vi "Calculate Galvo Control Voltage to Image Size and Max FOV.vi"(8 "Error In":errorcluster, 11 "System Parameters [In]":T1={"Optical /HW Parameters"={"Focal Length [mm]"=0.0, "Scan Lens EFL[mm]"=0.0, "Tube Lens EFL[mm]"=0.0, "Galvo V Range (+/-)"=0.0, "Galvo Max Half Angle [Deg]"=0.0, "Max Galvo Range[%]"=0.0}, "Vibratome"={"Z Bottom [mm]"=0.0, "Pre Cut Dwell [s]"=0.0, "Blade Frequency [RPM]"=0, "Slice Speed [mm/s]"=0.0, "Post Cut Dwell [s]"=0.0, "Ramp Time [s]"=0.0, "Start X [mm]"=0.0, "Start Y [mm]"=0.0, "Slice Length [mm]"=0.0, "Slice Axis"=enum."Y Axis", "Controller VISA Ref"="COM4"}, "Table Stages"={"X Stage"={"Position"=0.0, "Is.Enabled?"=FALSE, "Is.Connected?"=FALSE, "Device SN"="45876539", "AccelerationMaximum"=0.0, "VelocityMaximum"=0.0, "Acceleration"=0.0, "Velocity"=0.0, "waitTimeout (ms)"=0, "Model"=enum."None", "Is.Homed?"=FALSE}, "Y Stage"={"Position"=0.0, "Is.Enabled?"=FALSE, "Is.Connected?"=FALSE, "Device SN"="45876539", "AccelerationMaximum"=0.0, "VelocityMaximum"=0.0, "Acceleration"=0.0, "Velocity"=0.0, "waitTimeout (ms)"=0, "Model"=enum."None", "Is.Homed?"=FALSE}, "Z Stage"={"Position"=0.0, "Is.Enabled?"=FALSE, "Is.Connected?"=FALSE, "Device SN"="45876539", "AccelerationMaximum"=0.0, "VelocityMaximum"=0.0, "Acceleration"=0.0, "Velocity"=0.0, "waitTimeout (ms)"=0, "Model"=enum."None", "Is.Homed?"=FALSE}}, "Imaging Parameter"={"Raster Scan Direction"=enum."Uni Directional", "Pixel Dwell Time [Clock Cycles]"=0, "Flyback Time [Clock Cycles]"=0, "XY Center [um]"={"X"=1.0, "Y"=1.0}, "Pixel Step Size [um]"=1.0, "XY Image Resolution"=enum."256 x 256", "Custom"=FALSE, "Custom Size"={"X"=1, "Y"=1}, "Line Averages"=1}} {"Imaging Parameter"."Line Averages" min=1 max=30 step=1; "Imaging Parameter"."Flyback Time [Clock Cycles]" max=10 step=1; "Imaging Parameter"."Pixel Step Size [um]" min=0.0 max=10.0 step=0.01; "Imaging Parameter"."Custom Size"."Y" min=1 max=30 step=1; "Imaging Parameter"."Custom Size"."X" min=1 max=30 step=1; "Imaging Parameter"."XY Center [um]"."Y" min=1.0 max=30.0 step=1.0; "Imaging Parameter"."XY Center [um]"."X" min=1.0 max=30.0 step=1.0; "Imaging Parameter"."Pixel Dwell Time [Clock Cycles]" max=10 step=1}) -> (0 "Error Out":errorcluster, 1 "Max Half FOV (um)":dbl, 2 "Galvo [um/V]":dbl, 3 "System Parameters [Out]":T1={"Optical /HW Parameters"={"Focal Length [mm]"=0.0, "Scan Lens EFL[mm]"=0.0, "Tube Lens EFL[mm]"=0.0, "Galvo V Range (+/-)"=0.0, "Galvo Max Half Angle [Deg]"=0.0, "Max Galvo Range[%]"=0.0}, "Vibratome"={"Z Bottom [mm]"=0.0, "Pre Cut Dwell [s]"=0.0, "Blade Frequency [RPM]"=0, "Slice Speed [mm/s]"=0.0, "Post Cut Dwell [s]"=0.0, "Ramp Time [s]"=0.0, "Start X [mm]"=0.0, "Start Y [mm]"=0.0, "Slice Length [mm]"=0.0, "Slice Axis"=enum."Y Axis", "Controller VISA Ref"="COM4"}, "Table Stages"={"X Stage"={"Position"=0.0, "Is.Enabled?"=FALSE, "Is.Connected?"=FALSE, "Device SN"="45876539", "AccelerationMaximum"=0.0, "VelocityMaximum"=0.0, "Acceleration"=0.0, "Velocity"=0.0, "waitTimeout (ms)"=0, "Model"=enum."None", "Is.Homed?"=FALSE}, "Y Stage"={"Position"=0.0, "Is.Enabled?"=FALSE, "Is.Connected?"=FALSE, "Device SN"="45876539", "AccelerationMaximum"=0.0, "VelocityMaximum"=0.0, "Acceleration"=0.0, "Velocity"=0.0, "waitTimeout (ms)"=0, "Model"=enum."None", "Is.Homed?"=FALSE}, "Z Stage"={"Position"=0.0, "Is.Enabled?"=FALSE, "Is.Connected?"=FALSE, "Device SN"="45876539", "AccelerationMaximum"=0.0, "VelocityMaximum"=0.0, "Acceleration"=0.0, "Velocity"=0.0, "waitTimeout (ms)"=0, "Model"=enum."None", "Is.Homed?"=FALSE}}, "Imaging Parameter"={"Raster Scan Direction"=enum."Uni Directional", "Pixel Dwell Time [Clock Cycles]"=0, "Flyback Time [Clock Cycles]"=0, "XY Center [um]"={"X"=1.0, "Y"=1.0}, "Pixel Step Size [um]"=1.0, "XY Image Resolution"=enum."256 x 256", "Custom"=FALSE, "Custom Size"={"X"=1, "Y"=1}, "Line Averages"=1}} {"Imaging Parameter"."Line Averages" min=1 max=30 step=1; "Imaging Parameter"."Flyback Time [Clock Cycles]" max=10 step=1; "Imaging Parameter"."Pixel Step Size [um]" min=0.0 max=10.0 step=0.01; "Imaging Parameter"."Custom Size"."Y" min=1 max=30 step=1; "Imaging Parameter"."Custom Size"."X" min=1 max=30 step=1; "Imaging Parameter"."XY Center [um]"."Y" min=1.0 max=30.0 step=1.0; "Imaging Parameter"."XY Center [um]"."X" min=1.0 max=30.0 step=1.0; "Imaging Parameter"."Pixel Dwell Time [Clock Cycles]" max=10 step=1})   [LabVIEW 2018]
doc: "This is assuming 1:1 magnification between X and Y galvo\n\nChief Ray Angle : The chief ray angle at the back pupil of the objective for the galvo's maximum steering angle.\nOptical Mag: The optical magnification between the galvo and the objective's back pupil\nGalvo: The amount of motion in the object plane per V of control signal on the Galvo.\nMax Half FOV (um) : The maximum object height when the galvos are rotated to max angle."
uses:
  Controls/System Parameters.ctl
  Hardware/Table Stage/Controls/Translation Stage Cluster.ctl
  Controls/Translation Stage Types.ctl
  Controls/Scan Direction.ctl
panel:
  out "Chief Ray Angle":dbl
  out "Optical Mag":dbl
  # "X"
  # "X"
  # "X"
  # "X"
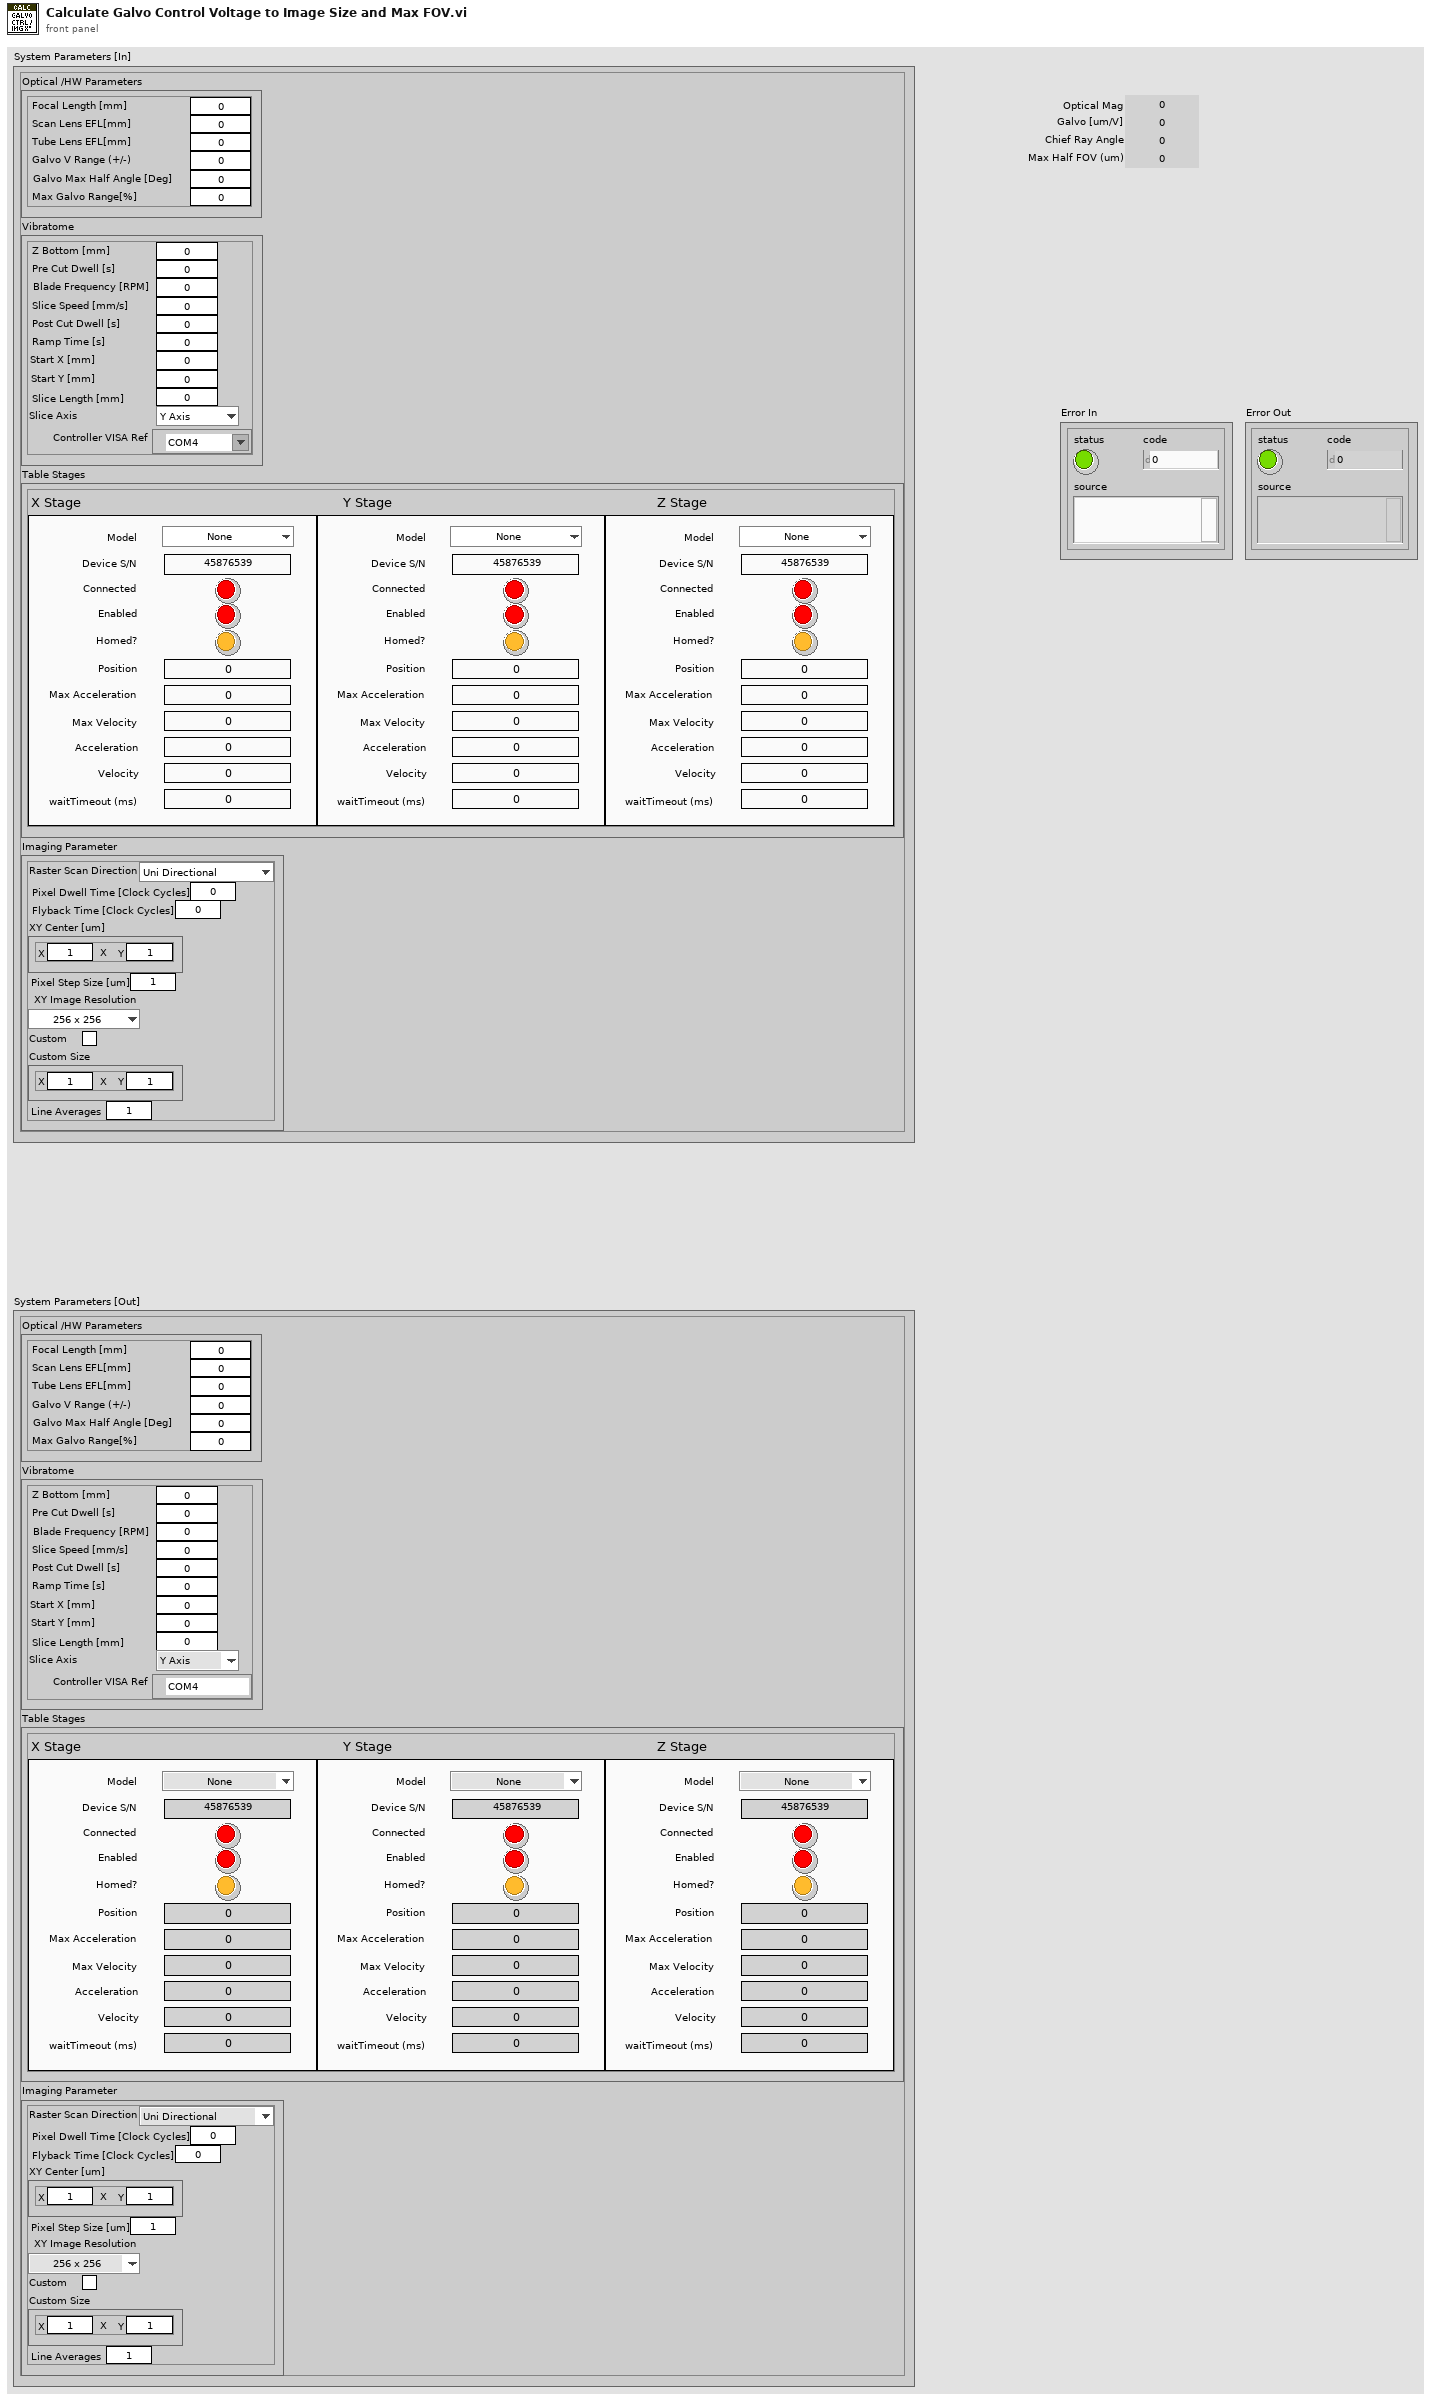
[diagram p1: front panel]
types:
  T1 = typedef "System Parameters.ctl" = cluster{"Optical /HW Parameters":cluster{"Focal Length [mm]":dbl, "Scan Lens EFL[mm]":dbl, "Tube Lens EFL[mm]":dbl, "Galvo V Range (+/-)":dbl, "Galvo Max Half Angle [Deg]":dbl, "Max Galvo Range[%]":dbl}, "Vibratome":cluster{"Z Bottom [mm]":dbl, "Pre Cut Dwell [s]":dbl, "Blade Frequency [RPM]":u16, "Slice Speed [mm/s]":dbl, "Post Cut Dwell [s]":dbl, "Ramp Time [s]":dbl, "Start X [mm]":dbl, "Start Y [mm]":dbl, "Slice Length [mm]":dbl, "Slice Axis":enum16{"X Axis", "Y Axis", "Z Axis"}, "Controller VISA Ref":refnum<visa-resource-name>}, "Table Stages":cluster{"X Stage":T2, "Y Stage":T2, "Z Stage":T2}, "Imaging Parameter":cluster{"Raster Scan Direction":T4, "Pixel Dwell Time [Clock Cycles]":u16, "Flyback Time [Clock Cycles]":u16, "XY Center [um]":cluster{"X":dbl, "Y":dbl}, "Pixel Step Size [um]":dbl, "XY Image Resolution":enum16{"32 x 32", "64 x 64", "128 x 128", "256 x 256", "512 x 512", "1024 x 1024", "2048 x 2048"}, "Custom":bool, "Custom Size":cluster{"X":u16, "Y":u16}, "Line Averages":u8}}
  T2 = typedef "Translation Stage Cluster.ctl" = cluster{"Position":dbl, "Is.Enabled?":bool, "Is.Connected?":bool, "Device SN":string, "AccelerationMaximum":dbl, "VelocityMaximum":dbl, "Acceleration":dbl, "Velocity":dbl, "waitTimeout (ms)":i32, "Model":T3, "Is.Homed?":bool}
  T3 = typedef "Translation Stage Types.ctl" = enum16{"None", "Thorlabs LTS", "Thorlabs MLJ"}
  T4 = typedef "Scan Direction.ctl" = enum16{"Uni Directional", "Bi Directional", "None"}
  T5 = cluster{"Focal Length [mm]":dbl, "Scan Lens EFL[mm]":dbl, "Tube Lens EFL[mm]":dbl, "Galvo V Range (+/-)":dbl, "Galvo Max Half Angle [Deg]":dbl, "Max Galvo Range[%]":dbl}
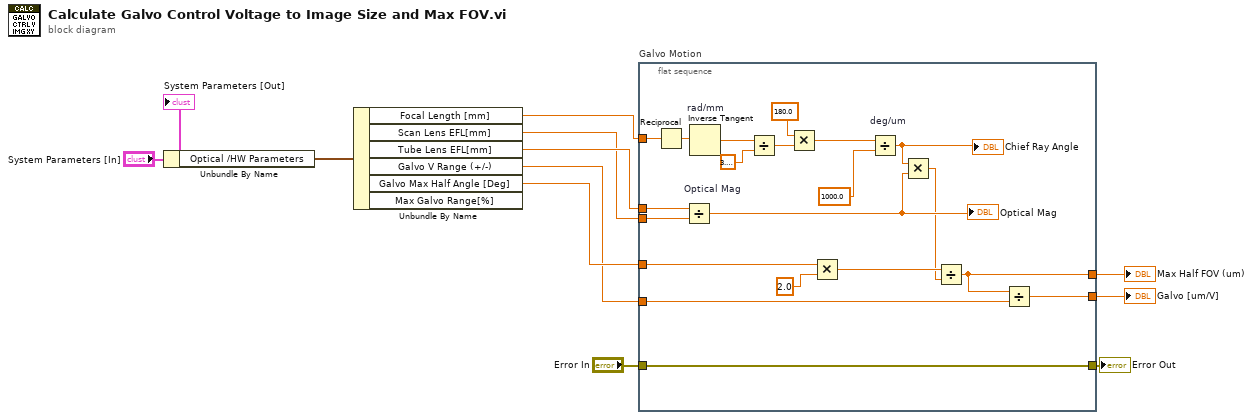
[diagram p0: block diagram]
diagram:
  n1 = Unbundle By Name("System Parameters [In]") -> ("Optical /HW Parameters"=w10:T5)
  n2 = Unbundle By Name(w10) -> ("Focal Length [mm]"=w7:dbl, "Scan Lens EFL[mm]"=w5:dbl, "Tube Lens EFL[mm]"=w6:dbl, "Galvo V Range (+/-)"=w8:dbl, "Galvo Max Half Angle [Deg]"=w9:dbl)  [unwired: 1 out]
  n3 = flat-sequence "Galvo Motion" {
    tunnel: w9 -> [w15]
    tunnel: w8 -> [w14]
    tunnel: w7 -> [w28]
    tunnel: w6 -> [w27]
    tunnel: w5 -> [w26]
    tunnel: "Error In" -> [w25]
    tunnel: [w25] -> w3
    tunnel: [w12] -> w2
    tunnel: [w13] -> w1
    frame #0 {
      n4 = Reciprocal(x=w28) -> (1/x=w29:dbl)
      n5 = Divide "Optical Mag"(x=w27, y=w26) -> (x/y=w18:dbl)
      "Optical Mag" <- w18
      n6 = Inverse Tangent "rad/mm"(1:w29) -> (0:w30:dbl)
      n7 = Divide(x=w30, y=3.141592653589793) -> (x/y=w24:dbl)
      n8 = Multiply(x=180.0, y=w24) -> (x*y=w20:dbl)
      n9 = Multiply(x=w15, y=2.0 ("x")) -> (x*y=w17:dbl)
      n10 = Divide "deg/um"(x=w20, y=1000.0) -> (x/y=w19:dbl)
      "Chief Ray Angle" <- w19
      n11 = Multiply(x=w19, y=w18) -> (x*y=w16:dbl)
      n12 = Divide(x=w17, y=w16) -> (x/y=w12:dbl)
      n13 = Divide(x=w12, y=w14) -> (x/y=w13:dbl)
    }
  }
  "Galvo [um/V]" <- w1
  "Max Half FOV (um)" <- w2
  "System Parameters [Out]" <- "System Parameters [In]"
  "Error Out" <- w3
